vi "Image to SGL Array.vi"(7 "Optional Rectangle":i32[](array[numeric]), 8 "error in (no error)":errorcluster, 11 "Image":T1) -> (0 "error out":errorcluster, 3 "Image Pixels (Float)":sgl[][](array[numeric]))   [LabVIEW 2021]
uses:
  <vilib>/vision/Image Controls.llb/IMAQ Image.ctl
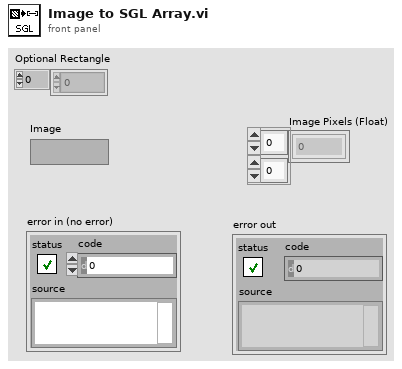
[diagram p1: front panel]
types:
  T1 = typedef "IMAQ Image.ctl" = refnum<image>
  T2 = typedef "Image Type" = u32
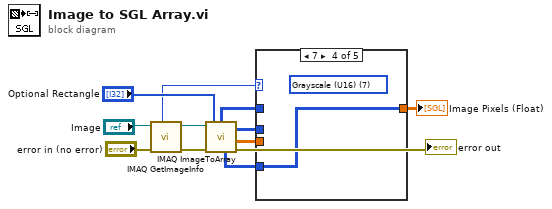
[diagram p0: block diagram]
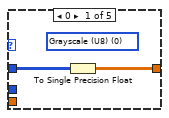
[diagram p2: hidden frame]
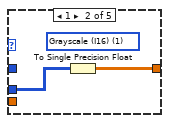
[diagram p3: hidden frame]
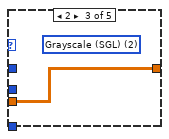
[diagram p4: hidden frame]
diagram:
  n1 = call "IMAQ GetImageInfo"("error in (no error)"="error in (no error)", "Image"="Image") -> ("error out"=w10:errorcluster, "Image Type"=w7:T2)  [unwired: 2 in, 6 out]
  n2 = call "IMAQ ImageToArray"("error in (no error)"=w10, "Optional Rectangle"="Optional Rectangle", "Image"="Image") -> ("Image Pixels (U16)"=w1:u16[][], "Image Pixels (Float)"=w4:sgl[][], "error out"=→"error out":errorcluster, "Image Pixels (U8)"=w6:u8[][], "Image Pixels (I16)"=w5:i16[][])  [unwired: 1 in]
  n3 = case shown="7" w7 {
    tunnel: w6 -> [w13 _ _ _ _]
    tunnel: [w12 w15 w16 w17 _] -> w2
    tunnel: w5 -> [_ w14 _ _ _]
    tunnel: w4 -> [_ _ w16 _ _]
    tunnel: w1 -> [_ _ _ w17 _]
    frame 0 {
      (unwired) T2 0 items=["Grayscale (U8)", "Grayscale (I16)", "Grayscale (SGL)", "Complex (CSG)", "RGB (U32)", "HSL (U32)", "RGB (U64)", "Grayscale (U16)"] ("Image Type")
      n4 = To Single Precision Float(number=w13) -> (single precision float=w12:sgl[][])
    }
    frame 1 {
      (unwired) T2 1 items=["Grayscale (U8)", "Grayscale (I16)", "Grayscale (SGL)", "Complex (CSG)", "RGB (U32)", "HSL (U32)", "RGB (U64)", "Grayscale (U16)"] ("Image Type")
      n5 = To Single Precision Float(number=w14) -> (single precision float=w15:sgl[][])
    }
    frame 2 {
      (unwired) T2 2 items=["Grayscale (U8)", "Grayscale (I16)", "Grayscale (SGL)", "Complex (CSG)", "RGB (U32)", "HSL (U32)", "RGB (U64)", "Grayscale (U16)"] ("Image Type")
    }
    frame 7 {
      (unwired) T2 7 items=["Grayscale (U8)", "Grayscale (I16)", "Grayscale (SGL)", "Complex (CSG)", "RGB (U32)", "HSL (U32)", "RGB (U64)", "Grayscale (U16)"] ("Image Type")
    }
    frame 3, Default {
    }
  }
  "Image Pixels (Float)" <- w2
